vi "Get Packed Library Name.vi"(11 "Plugin Configuration in":refnum<class "Plugin Configuration.lvclass">) -> (2 "packed library name":string, 3 "Plugin Configuration out":refnum<class "Plugin Configuration.lvclass">)   [LabVIEW 2017, in "DSF Core.lvlib" / "Plugin Configuration.lvclass"]
uses:
  Plugin Configuration.lvclass
  Plugin Configuration.lvclass/Plugin Configuration.ctl
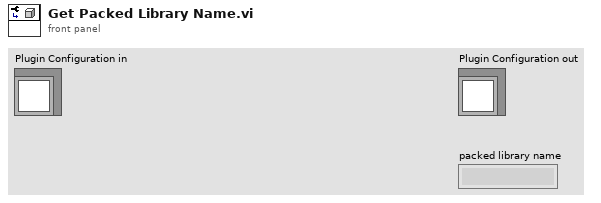
[diagram p1: front panel]
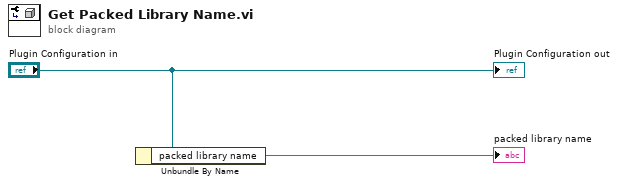
[diagram p0: block diagram]
diagram:
  n1 = Unbundle By Name("Plugin Configuration in") -> ("packed library name"=→"packed library name":string)
  "Plugin Configuration out" <- "Plugin Configuration in"
